vi "4155C Sample Config SMUs FPP v3.1.vi"(2 "FPP - Probe 2":u32(ring)=3 items=["SMU1  ", "SMU2  ", "SMU3  ", "SMU4  ", "SMU5  ", "SMU6  ", "VSU1  ", "VSU2  "], 4 "FPP - Probe 1":u32(ring) items=["SMU1  ", "SMU2  ", "SMU3  ", "SMU4  ", "SMU5  ", "SMU6  ", "VSU1  ", "VSU2  "], 5 "FPP - Drain":u32(ring)=1 items=["SMU1  ", "SMU2  ", "SMU3  ", "SMU4  ", "SMU5  ", "SMU6  ", "VSU1  ", "VSU2  "], 6 "FPP - Gate":u32(ring)=2 items=["SMU1  ", "SMU2  ", "SMU3  ", "SMU4  ", "SMU5  ", "SMU6  ", "VSU1  ", "VSU2  "], 7 "FPP - Source":u32(ring)=6 items=["SMU1  ", "SMU2  ", "SMU3  ", "SMU4  ", "SMU5  ", "SMU6  ", "VSU1  ", "VSU2  "], 8 "error in (no error)":errorcluster, 9 "Drain Standby":bool, 10 "Gate Standby":bool, 11 "VISA resource name in":refnum<visa-resource-name>) -> (0 "error out":errorcluster, 3 "VISA Resource Name out":refnum<visa-resource-name>)   [LabVIEW 2016]
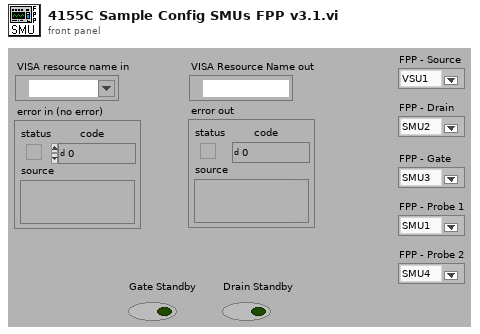
[diagram p1: front panel]
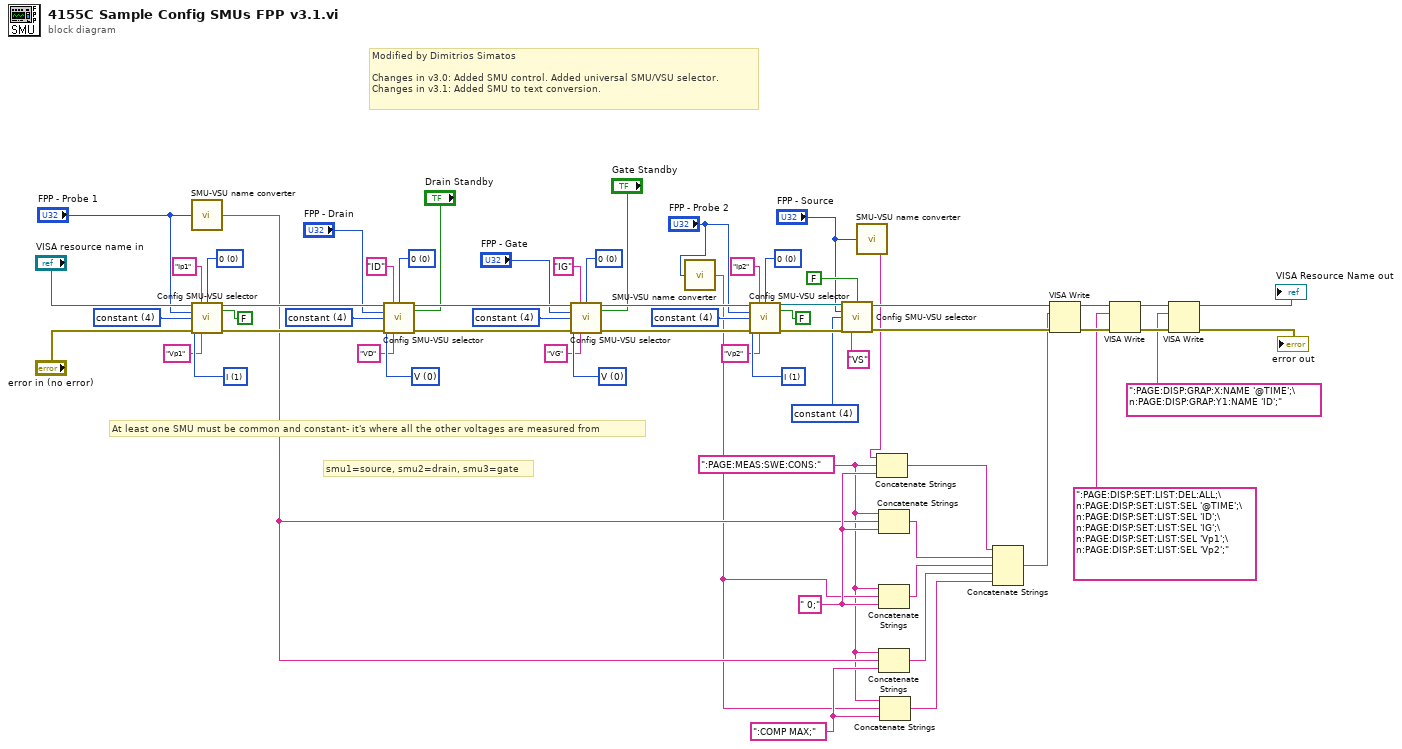
[diagram p0: block diagram]
diagram:
  w6 = ":COMP MAX;" ("write buffer (\"\")")
  w8 = " 0;" ("write buffer (\"\")")
  w3 = ":PAGE:MEAS:SWE:CONS:" ("write buffer (\"\")")
  w32 = u32 4 items=["disabled  ", "VAR1  ", "VAR2  ", "VAR1'  ", "constant  "] ("function")
  w43 = u32 1 items=["V  ", "I  ", "V pulse  ", "I pulse  ", "  common  "] ("mode")
  w44 = u32 0 items=["0  ", "10K Ohms  ", "100K Ohms  ", "1M Ohms  "] ("series resistance *")
  w46 = u32 4 items=["disabled  ", "VAR1  ", "VAR2  ", "VAR1'  ", "constant  "] ("function")
  w48 = u32 0 items=["V  ", "I  ", "V pulse  ", "I pulse  ", "  common  "] ("mode")
  w49 = u32 0 items=["0  ", "10K Ohms  ", "100K Ohms  ", "1M Ohms  "] ("series resistance *")
  w51 = u32 4 items=["disabled  ", "VAR1  ", "VAR2  ", "VAR1'  ", "constant  "] ("function")
  w53 = u32 0 items=["V  ", "I  ", "V pulse  ", "I pulse  ", "  common  "] ("mode")
  w54 = u32 0 items=["0  ", "10K Ohms  ", "100K Ohms  ", "1M Ohms  "] ("series resistance *")
  w56 = u32 4 items=["disabled  ", "VAR1  ", "VAR2  ", "VAR1'  ", "constant  "] ("function")
  w59 = u32 1 items=["V  ", "I  ", "V pulse  ", "I pulse  ", "  common  "] ("mode")
  w60 = u32 0 items=["0  ", "10K Ohms  ", "100K Ohms  ", "1M Ohms  "] ("series resistance *")
  w62 = u32 4 items=["disabled  ", "VAR1  ", "VAR2  ", "VAR1'  ", "constant  "] ("function")
  # "Modified by Dimitrios Simatos\n\nChanges in v3.0: Added SMU control. Added universal SMU/VSU selector.\nChanges in v3.1: Added SMU to text conversion."
  # "smu1=source, smu2=drain, smu3=gate"
  # "At least one SMU must be common and constant- it's where all the other voltages are measured from"
  n1 = call "SMU-VSU name converter.vi"("unit to configure"="FPP - Probe 1") -> ("SMU/VSU to be configured"=w5:string)
  n2 = call "Config SMU-VSU selector.vi"("VISA session"="VISA resource name in", "I name (max 6 chars)"="Ip1", "standby"=FALSE, "unit to configure"="FPP - Probe 1", "function"=w62, "mode"=w59, "error in (no error)"="error in (no error)", "V name (max 6 chars)"="Vp1", "series resistance *"=w60) -> ("dup VISA resource name"=w40:refnum<visa-resource-name>, "error out"=w39:errorcluster)  [unwired: 3 in, 2 out]
  n3 = call "Config SMU-VSU selector.vi"("VISA session"=w40, "I name (max 6 chars)"="ID", "standby"="Drain Standby", "unit to configure"="FPP - Drain", "function"=w56, "mode"=w53, "error in (no error)"=w39, "V name (max 6 chars)"="VD", "series resistance *"=w54) -> ("dup VISA resource name"=w37:refnum<visa-resource-name>, "error out"=w38:errorcluster)  [unwired: 3 in, 2 out]
  n4 = call "Config SMU-VSU selector.vi"("VISA session"=w37, "I name (max 6 chars)"="IG", "standby"="Gate Standby", "unit to configure"="FPP - Gate", "function"=w51, "mode"=w48, "error in (no error)"=w38, "V name (max 6 chars)"="VG", "series resistance *"=w49) -> ("dup VISA resource name"=w36:refnum<visa-resource-name>, "error out"=w35:errorcluster)  [unwired: 3 in, 2 out]
  n5 = call "SMU-VSU name converter.vi"("unit to configure"="FPP - Probe 2") -> ("SMU/VSU to be configured"=w4:string)
  n6 = call "Config SMU-VSU selector.vi"("VISA session"=w36, "I name (max 6 chars)"="Ip2", "standby"=FALSE, "unit to configure"="FPP - Probe 2", "function"=w46, "mode"=w43, "error in (no error)"=w35, "V name (max 6 chars)"="Vp2", "series resistance *"=w44) -> ("dup VISA resource name"=w30:refnum<visa-resource-name>, "error out"=w34:errorcluster)  [unwired: 3 in, 2 out]
  n7 = call "Config SMU-VSU selector.vi"("VISA session"=w30, "standby"=FALSE, "unit to configure"="FPP - Source", "function"=w32, "error in (no error)"=w34, "V name (max 6 chars)"="VS") -> ("dup VISA resource name"=w28:refnum<visa-resource-name>, "error out"=w29:errorcluster)  [unwired: 6 in, 2 out]
  n8 = call "SMU-VSU name converter.vi"("unit to configure"="FPP - Source") -> ("SMU/VSU to be configured"=w14:string)
  n9 = Concatenate Strings(w14, w3, w8) -> (w12:string)
  n10 = Concatenate Strings(w3, w5, w8) -> (w10:string)
  n11 = Concatenate Strings(w3, w4, w8) -> (w7:string)
  n12 = Concatenate Strings(w3, w5, w6) -> (w2:string)
  n13 = Concatenate Strings(w3, w4, w6) -> (w1:string)
  n14 = Concatenate Strings(w12, w10, w7, w2, w1) -> (w13:string)
  n15 = VISA Write(VISA resource name=w28, write buffer=w13, error in (no error)=w29) -> (VISA resource name out=w27:refnum<visa-resource-name>, error out=w22:errorcluster)  [unwired: 1 out]
  n16 = VISA Write(VISA resource name=w27, write buffer=":PAGE:DISP:SET:LIST:DEL:ALL;\n:PAGE:DISP:SET:LIST:SEL '@TIME';\n:PAGE:DISP:SET:LIST:SEL 'ID';\n:PAGE:DISP:SET:LIST:SEL 'IG';\n:PAGE:DISP:SET:LIST:SEL 'Vp1';\n:PAGE:DISP:SET:LIST:SEL 'Vp2';" ("write buffer (\"\")"), error in (no error)=w22) -> (VISA resource name out=w26:refnum<visa-resource-name>, error out=w23:errorcluster)  [unwired: 1 out]
  n17 = VISA Write(VISA resource name=w26, write buffer=":PAGE:DISP:GRAP:X:NAME '@TIME';\n:PAGE:DISP:GRAP:Y1:NAME 'ID';" ("write buffer (\"\")"), error in (no error)=w23) -> (VISA resource name out=→"VISA Resource Name out":refnum<visa-resource-name>, error out=→"error out":errorcluster)  [unwired: 1 out]
